vi "DatabaseUpdate.vi"(3 "Input":string, 8 "error in (no error)":errorcluster, 11 "Imie":string) -> (0 "error out":errorcluster)   [LabVIEW 2024]
uses:
  <vilib>/addons/database/Connection.llb/DB Tools Open Connec (Path).vi
  <vilib>/addons/database/_DB Variant To Data/Database Variant To Data.xnode
  <vilib>/addons/database/NI_Database_API.lvlib
panel:
  out "s? t:f":i32
  out "Kolumna 2 czyli input":string
  out "Final Data":string[][](array[string])
  out "Initial Data":string[][](array[string])
  # "Numer wiersza"
  # "Nazwa kolumny"
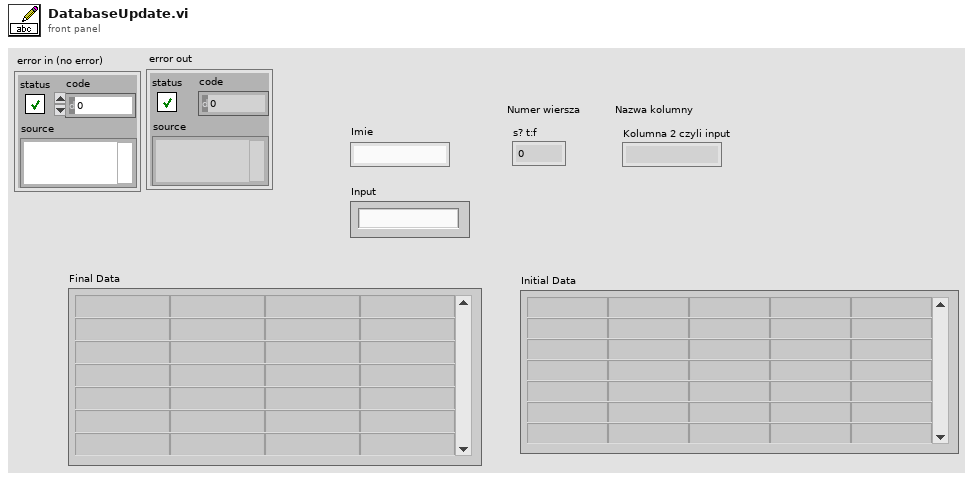
[diagram p1: front panel]
types:
  T1 = typedef "NI_Database_API.lvlib/Conn ObjectReference.ctl" = refnum<k1>
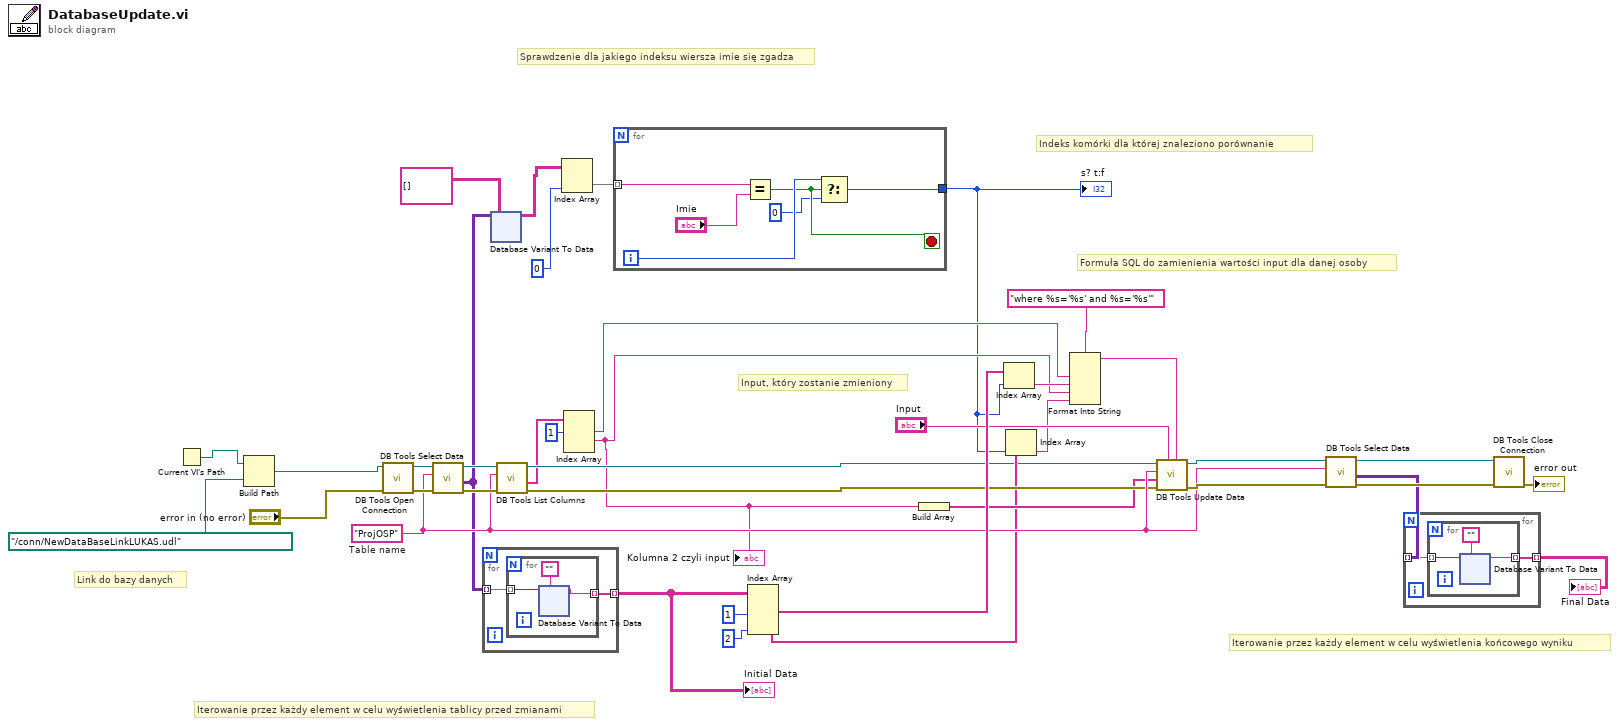
[diagram p0: block diagram]
diagram:
  w25 = "ProjOSP"  # Table name
  # "Iterowanie przez każdy element w celu wyświetlenia tablicy przed zmianami"
  # "Iterowanie przez każdy element w celu wyświetlenia końcowego wyniku"
  # "Formuła SQL do zamienienia wartości input dla danej osoby"
  # "Input, który zostanie zmieniony"
  # "Sprawdzenie dla jakiego indeksu wiersza imie się zgadza"
  # "Link do bazy danych"
  # "Indeks komórki dla której znaleziono porównanie"
  n1 = Current VI's Path() -> (path=w39:path)
  n2 = Build Path(base path=w39, name or relative path=path "../conn/NewDataBaseLinkLUKAS.udl") -> (appended path=w11:path)
  n3 = call-poly <vilib>:"DB Tools Open Connection.vi"("error in (no error)"="error in (no error)", "connection information"=w11) -> ("error out"=w36:errorcluster, "connection reference"=w37:T1)  [unwired: 6 in]
  n4 = call <vilib>:"DB Tools Select Data.vi"("error in (no error)"=w36, "table"=w25, "connection reference"=w37) -> ("error out"=w26:errorcluster, "data"=w6:variant[][], "connection reference out"=w27:T1)  [unwired: 3 in]
  n5 = for {
    tunnel: w6 -> [w41] mode=indexing
    tunnel: [w40] -> w21 mode=indexing
    n6 = for {
      tunnel: w41 -> [w43] mode=indexing
      tunnel: [w42] -> w40 mode=indexing
      n7 = xnode "Database Variant To Data"("database variant"=w43, "type"="") -> ("data"=w42:string)  [unwired: 1 in, 1 out]
    }
  }
  "Initial Data" <- w21
  n8 = xnode "Database Variant To Data"("database variant"=w6, "type"=string[][] []) -> ("data"=w4:string[][])  [unwired: 1 in, 1 out]
  n9 = call <vilib>:"DB Tools List Columns.vi"("error in (no error)"=w26, "table"=w25, "connection reference"=w27) -> ("error out"=w23:errorcluster, "columns"=w7:string[], "connection reference out"=w12:T1)  [unwired: 1 in, 1 out]
  n10 = Index Array(array=w4, index (col)=0 ("disabled index (col)")) -> (element=w2:string[])  [unwired: 1 in]
  n11 = Index Array(array=w7, index #1=1 ("disabled index (col)")) -> (element #1=w16:string, element #2=w10:string)  [unwired: 2 in, 1 out]
  "Kolumna 2 czyli input" <- w10
  n12 = for {
    tunnel: w2 -> [w80] mode=indexing
    tunnel: [w78] -> w1
    i -> [w81]
    stop <- w79 stop-if-true
    n13 = Equal?(x=w80, y="Imie") -> (x = y?=w79:bool)
    n14 = Select(t=w81, s=w79, f=0) -> (s? t:f=w78:i32)
  }
  "s? t:f" <- w1
  n15 = Index Array(array=w21, index (col) #1=1 ("disabled index (col)"), index (col) #2=2 ("index (col)")) -> (element #1=w28:string[], element #2=w18:string[])  [unwired: 2 in]
  n16 = Build Array(w10) -> (w22:string[])
  n17 = Index Array(array=w28, index=w1) -> (element=w15:string)
  n18 = Index Array(array=w18, index=w1) -> (element=w14:string)
  n19 = Format Into String(format string="where %s='%s' and %s='%s'", w16, w15, w10, w14) -> (resulting string=w13:string)  [unwired: 2 in, 1 out]
  n20 = call <vilib>:"DB Tools Update Data.vi"("condition"=w13, "data"="Input", "error in (no error)"=w23, "columns"=w22, "table"=w25, "connection reference"=w12) -> ("error out"=w32:errorcluster, "connection reference out"=w33:T1)  [unwired: 4 in]
  n21 = call <vilib>:"DB Tools Select Data.vi"("error in (no error)"=w32, "table"=w25, "connection reference"=w33) -> ("error out"=w30:errorcluster, "data"=w29:variant[][], "connection reference out"=w31:T1)  [unwired: 3 in]
  n22 = for {
    tunnel: w29 -> [w84] mode=indexing
    tunnel: [w83] -> w20 mode=indexing
    n23 = for {
      tunnel: w84 -> [w86] mode=indexing
      tunnel: [w85] -> w83 mode=indexing
      n24 = xnode "Database Variant To Data"("database variant"=w86, "type"="") -> ("data"=w85:string)  [unwired: 1 in, 1 out]
    }
  }
  "Final Data" <- w20
  n25 = call <vilib>:"DB Tools Close Connection.vi"("error in (no error)"=w30, "connection reference"=w31) -> ("error out"=→"error out":errorcluster)  [unwired: 5 in]
